vi "Read Com_Set.vi"(8 "error in (no error)":errorcluster, 11 "TCP In":refnum<class "TCP.lvclass">) -> (0 "error out":errorcluster, 2 "Com_Set":T1, 3 "TCP Out":refnum<class "TCP.lvclass">)   [LabVIEW 2019, in "TCP.lvclass"]
uses:
  TCP.lvclass
  SettingCtrl.ctl
  TCP.lvclass/TCP.ctl
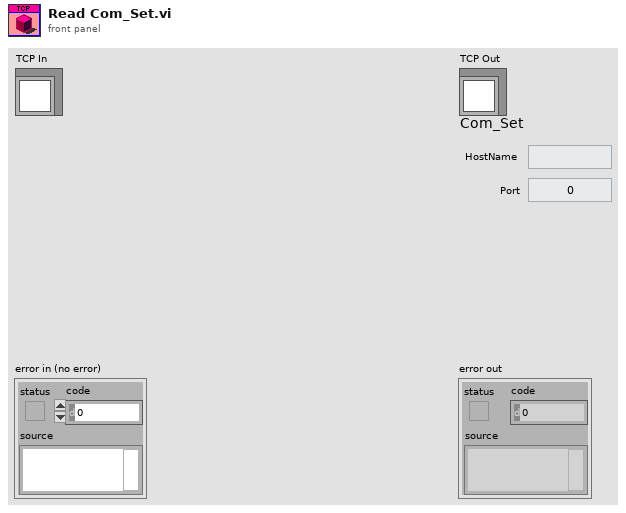
[diagram p1: front panel]
types:
  T1 = typedef "TCP.lvclass/SettingCtrl.ctl" = cluster{"HostName":string, "Port":u16}
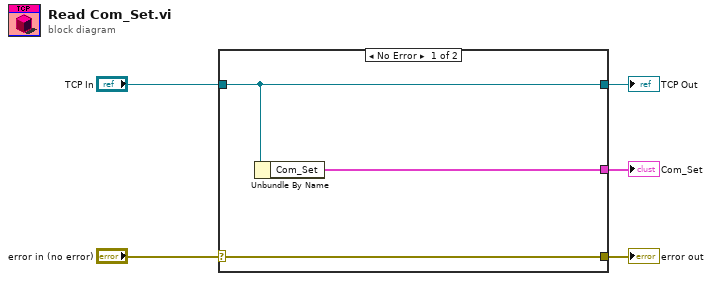
[diagram p0: block diagram]
diagram:
  n1 = case shown="No Error" "error in (no error)" {
    selector: "error in (no error)" -> [w8 w9]
    tunnel: [w8 w9] -> w4
    tunnel: [w7 w10] -> w2
    tunnel: "TCP In" -> [w7 w10]
    tunnel: [w6 _] -> w1
    frame No Error {
      n2 = Unbundle By Name(w7) -> ("Com_Set"=w6:T1)
    }
    frame Error {
    }
  }
  "error out" <- w4
  "TCP Out" <- w2
  "Com_Set" <- w1
